vi "PXI-Enumerate AI Channels.vi"() -> (3 "AI.PhysicalChans":tag[](array[tag]))   [LabVIEW 2020]
uses:
  <resource>/objmgr/daqmx.rc
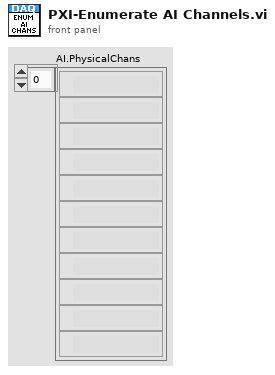
[diagram p1: front panel]
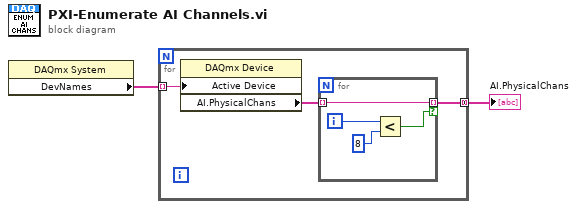
[diagram p0: block diagram]
diagram:
  n1 = property class="DAQmx System"() -> ("DevNames"=w1:tag[])  [unwired: 2 in, 2 out]
  n2 = for {
    tunnel: w1 -> [w5] mode=indexing
    tunnel: [w3] -> w2 mode=concatenating
    n3 = property class="DAQmx Device"("Active Device"=w5) -> ("AI.PhysicalChans"=w4:tag[])  [unwired: 2 in, 2 out]
    n4 = for {
      tunnel: w4 -> [w7] mode=indexing
      tunnel: [w7] -> w3 mode=indexing if=w6
      i -> [w8]
      n5 = Less?(x=w8, y=8) -> (x < y?=w6:bool)
    }
  }
  "AI.PhysicalChans" <- w2
